vi "Test harness - Is dependency.vi"(11 "Type of file to test":T1=".vi") -> (0 "error out":errorcluster, 3 "Is dependency":bool)   [LabVIEW 2021]
uses:
  Test harness file type.ctl
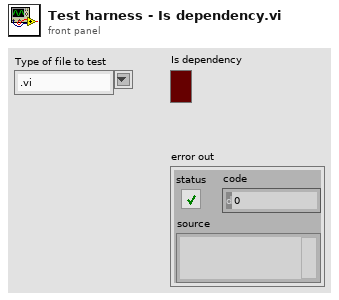
[diagram p1: front panel]
types:
  T1 = typedef "Test harness file type.ctl" = string
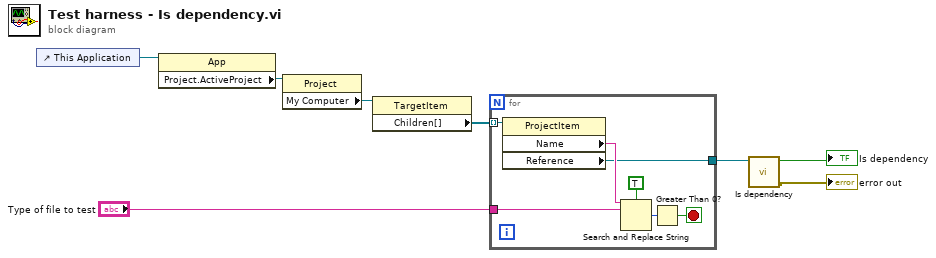
[diagram p0: block diagram]
diagram:
  n1 = control-ref of="This Application"() -> (w6:refnum<vi>)
  n2 = property class="App"(reference=w6) -> ("Project.ActiveProject"=w8:refnum<vi>)  [unwired: 1 in, 2 out]
  n3 = property class="Project"(reference=w8) -> ("My Computer"=w1:refnum<vi>)  [unwired: 1 in, 2 out]
  n4 = property class="TargetItem"(reference=w1) -> ("Children[]"=w7:refnum<vi>[])  [unwired: 1 in, 2 out]
  n5 = for {
    tunnel: w7 -> [w15] mode=indexing
    tunnel: [w11] -> w4
    tunnel: "Type of file to test" -> [w9]
    stop <- w12 stop-if-true
    n6 = property class="ProjectItem"(reference=w15) -> ("Name"=w13:string, "Reference"=w11:refnum<vi>)  [unwired: 1 in, 2 out]
    n7 = Search and Replace String(case sensitive?=TRUE ("ignore case? (F)"), input string=w13, search string=w9) -> (number of replacements=w10:i32)  [unwired: 5 in, 3 out]
    n8 = Greater Than 0?(x=w10) -> (x > 0?=w12:bool)
  }
  n9 = call "Is dependency.vi"("VI Reference"=w4) -> ("error out"=→"error out":errorcluster, "Is project dependency"=→"Is dependency":bool)  [unwired: 9 in]
